vi "dispose server listener.vi"(8 "error in":errorcluster, 11 "lvlibretls server listener in":refnum<class "lvlibretls server listener.lvclass">) -> (0 "error out":errorcluster)   [LabVIEW 2016, in "lvlibretls server listener.lvclass"]
uses:
  lvlibretls server listener.lvclass
  C:/Users/IEUser/Desktop/tlssimple/libretls/context parent/lvlibretls configurable context.lvclass
  lvlibretls server listener.lvclass/lvlibretls server listener.ctl
  context parent/lvlibretls configurable context.lvclass
  lv tls dll.lvlib
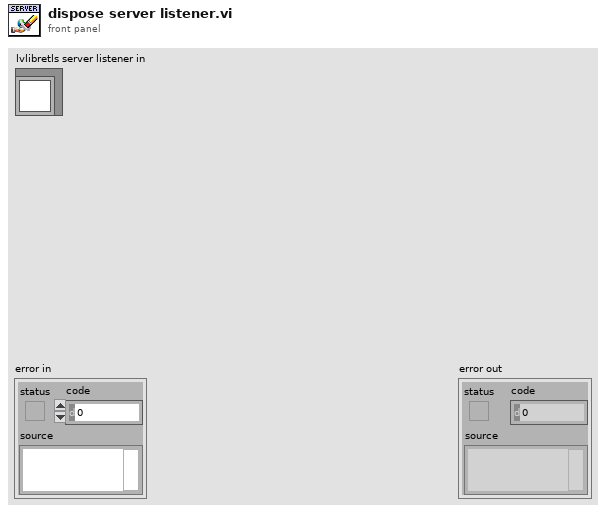
[diagram p1: front panel]
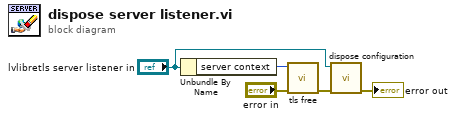
[diagram p0: block diagram]
diagram:
  n1 = Unbundle By Name("lvlibretls server listener in") -> ("server context"=w1:u64)
  n2 = call "tls free.vi"("error in"="error in", "tls context"=w1) -> ("error out"=w3:errorcluster)  [unwired: 9 in]
  n3 = call "dispose configuration.vi"("error in"=w3, "lvlibretls configurable context in"="lvlibretls server listener in") -> ("error out"=→"error out":errorcluster)  [unwired: 9 in]
